vi "List Classes in PPL.vi"(8 "error in":errorcluster, 11 "PPL Path":path) -> (0 "error out":errorcluster, 2 "Class Path Array":path[](array[path]), 3 "Class Name Array":string[](array[string]))   [LabVIEW 2019, in "ClassLoader.lvlib"]
doc: "Obtain Paths and Names for all classes contained in a PPL."
uses:
  ClassLoader.lvlib
  <vilib>/Utility/LVLibp/NI_PackedLibraryUtility.lvlib
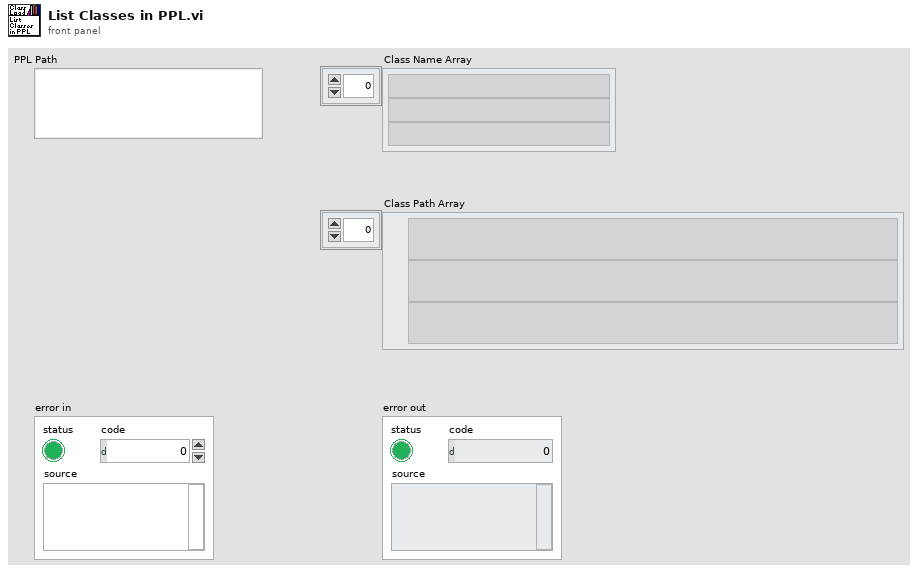
[diagram p1: front panel]
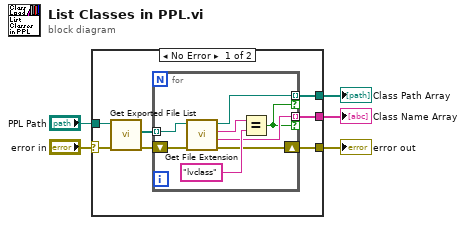
[diagram p0: block diagram]
diagram:
  n1 = case shown="No Error" "error in" {
    selector: "error in" -> [w11 _]
    tunnel: "PPL Path" -> [w12 _]
    tunnel: [w8 _] -> w3
    tunnel: [w7 _] -> w2
    tunnel: [w6 _] -> w1
    frame No Error {
      n2 = call <vilib>:"Get Exported File List.vi"("error in (no error)"=w11, "packed library path"=w12) -> ("error out"=w9:errorcluster, "paths"=w10:path[])  [unwired: 7 in, 1 out]
      n3 = for {
        tunnel: w10 -> [w19] mode=indexing
        shift-right: [w17] -> w8
        shift-left: w9 -> [w18]
        tunnel: [w16] -> w7 mode=indexing if=w14
        tunnel: [w15] -> w6 mode=indexing if=w14
        n4 = call <vilib>:"Get File Extension.vi"("error in (no error)"=w18, "file"=w19) -> ("error out"=w17:errorcluster, "filename without extension"=w15:string, "lowercase file extension"=w13:string, "dup file"=w16:path)  [unwired: 5 in, 1 out]
        n5 = Equal?(x=w13, y="lvclass" ("x")) -> (x = y?=w14:bool)
      }
    }
    frame Error {
    }
  }
  "error out" <- w3
  "Class Path Array" <- w2
  "Class Name Array" <- w1
